vi "Validate User Credentials.vi"(0 "iUser Configuration Manager DVR":refnum<data-value>, 5 "Username":string, 7 "Password":string, 11 "error in":errorcluster) -> (4 "dup iUser Configuration Manager DVR":refnum<data-value>, 6 "User Found":bool, 8 "Verified":bool, 10 "Verification Message":string, 15 "error out":errorcluster)   [LabVIEW 2020, in "User Configuration Manager.lvlib" / "By Ref.lvlib"]
doc: "Verifies the credentials of the user specified by user name."
uses:
  <vilib>/gpm_packages/@cs/user-manager/Source/User Configuration Manager Ref/By Ref.lvlib
  <vilib>/gpm_packages/@cs/user-manager/Source/iUser Configuration Manager/iUser Configuration Manager.lvclass
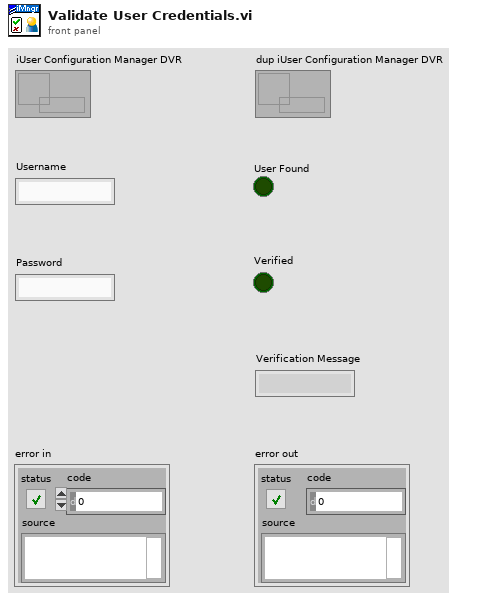
[diagram p1: front panel]
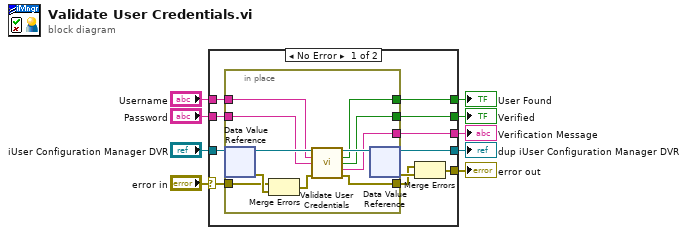
[diagram p0: block diagram]
diagram:
  n1 = case shown="No Error" "error in" {
    selector: "error in" -> [w18 w33]
    tunnel: "iUser Configuration Manager DVR" -> [w20 w32]
    tunnel: [w19 w33] -> w8
    tunnel: [w15 w32] -> w6
    tunnel: "Username" -> [w14 _]
    tunnel: "Password" -> [w13 _]
    tunnel: [w12 _] -> w3
    tunnel: [w11 _] -> w2
    tunnel: [w10 _] -> w1
    frame No Error {
      n2 = in-place "IPES" {
        in-place-border: [w24] -> w16
        in-place-border: w18 -> [w30]
        in-place-border: w14 -> [w23]
        in-place-border: w13 -> [w21]
        in-place-border: [w27] -> w12
        in-place-border: [w26] -> w11
        in-place-border: [w25] -> w10
        n3 = in-place-dvr #1(w20) -> (w29:refnum<class "iUser Configuration Manager.lvclass">, w31:errorcluster)
        n4 = Merge Errors(w30, w31) -> (w22:errorcluster)
        n5 = call-dynamic "Validate User Credentials.vi"("iUser Configuration Manager in"=w29, "Username"=w23, "Password"=w21, "error in (no error)"=w22) -> ("iUser Configuration Manager out"=w28:refnum<class "iUser Configuration Manager.lvclass">, "User Found"=w27:bool, "Verified"=w26:bool, "Verification Message"=w25:string, "error out"=w24:errorcluster)  [unwired: 7 in]
        n6 = in-place-dvr #1(w28) -> (w15:refnum<data-value>, w17:errorcluster)
      }
      n7 = Merge Errors(w16, w17) -> (w19:errorcluster)
    }
    frame Error {
    }
  }
  "error out" <- w8
  "dup iUser Configuration Manager DVR" <- w6
  "User Found" <- w3
  "Verified" <- w2
  "Verification Message" <- w1
